vi "Scan Initilize_BU.vi"(4 "Enable DMM Relay":bool=TRUE, 6 "Measure Maximun Voltage":dbl=100.0 format="%#_13g", 7 "Scan Measure\nTime":dbl=17.0, 8 "error in (no error)":errorcluster, 9 "Current Setting":u8[](array[numeric]), 10 "Channel Count":i32, 11 "VISA Refnum in":refnum<visa-resource-name>) -> (0 "error out":errorcluster, 1 "N channel number":i32, 2 "P channel number":i32, 3 "VISA Refnum out":refnum<visa-resource-name>)   [LabVIEW 2023]
uses:
  <instrlib>/Agilent 3446X Series/Agilent 3446X Series.lvlib
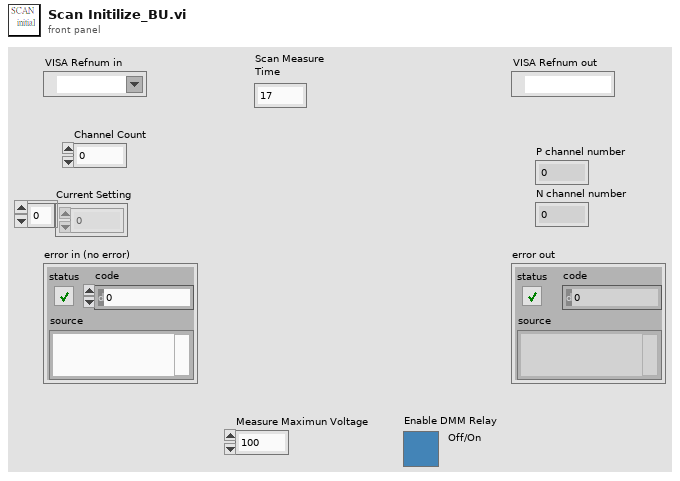
[diagram p1: front panel]
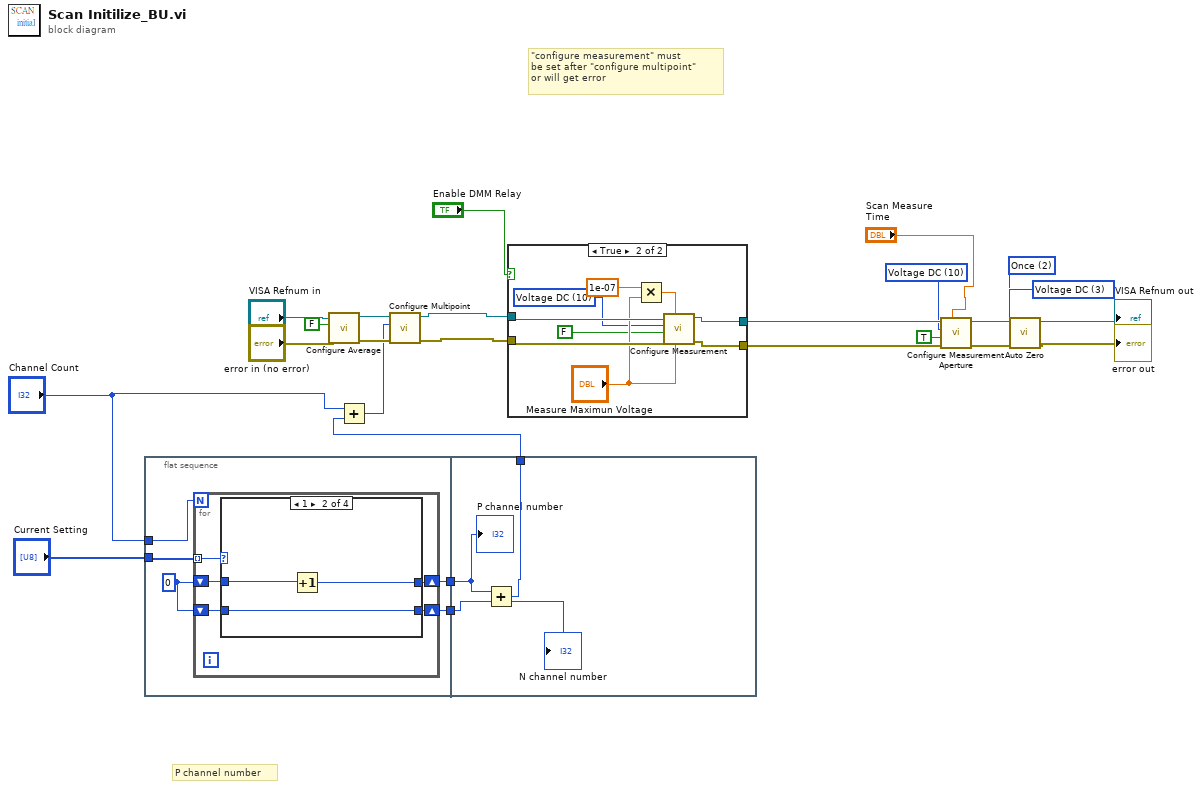
[diagram p0: block diagram]
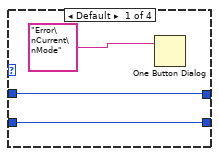
[diagram p3: hidden frame]
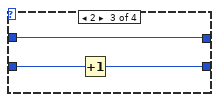
[diagram p4: hidden frame]
diagram:
  w12 = 3 items=["Current DC", "Resistance", "Temperature", "Voltage DC"] ("Zero Type (0: Current DC)")
  w11 = 2 items=["Disable", "Enable", "Once"] ("Auto Zero (1: Enable)")
  w9 = 10 items=["Continuity", "Current AC", "Current DC", "Diode", "Frequency", "Resistance 4-wire", "Period", "Resistance 2-wire", "Temperature", "Voltage AC", "Voltage DC", "Voltage DC Ratio", "Capacitance"] ("Measurement Function (0: Continuity)")
  # "P channel number"
  # "\"configure measurement\" must \nbe set after \"configure multipoint\"\nor will get error"
  n1 = flat-sequence {
    tunnel: "Channel Count" -> [w30]
    tunnel: "Current Setting" -> [w29]
    tunnel: [w27] -> w7
    tunnel: [w26] -> w6
    tunnel: w7 -> [w49]
    tunnel: w6 -> [w48]
    tunnel: [w47] -> w5
    frame #0 {
      w28 = 0 ("P_current_count")
      n2 = for {
        N: w30 -> [_]
        tunnel: w29 -> [w35] mode=indexing
        shift-right: [w33] -> w27
        shift-left: w28 -> [w34]
        shift-right: [w31] -> w26
        shift-left: w28 -> [w32]
        n3 = case shown="1" w35 {
          tunnel: w34 -> [w37 w41 w42 w46]
          tunnel: [w37 w40 w42 w46] -> w33
          tunnel: w32 -> [w36 w39 w44 w45]
          tunnel: [w36 w39 w43 w45] -> w31
          frame Default {
            n4 = One Button Dialog(message="Error\nCurrent\nMode" ("error source (\" \")")) -> ()  [unwired: 1 in, 1 out]
          }
          frame 1 {
            n5 = Increment(x=w41) -> (x+1=w40:i32)
          }
          frame 2 {
            n6 = Increment(x=w44) -> (x+1=w43:i32)
          }
          frame 0 {
          }
        }
      }
    }
    frame #1 {
      n7 = Add(x=w49, y=w48) -> (x+y=w47:i32)
      "P channel number" <- w49
      "N channel number" <- w48
    }
  }
  n8 = call <instrlib>:"Configure Average.vi"("error in (no error)"="error in (no error)", "Enable Statistics (F: Disable)"=FALSE, "VISA resource name"="VISA Refnum in") -> ("error out"=w19:errorcluster, "VISA resource name out"=w18:refnum<visa-resource-name>)  [unwired: 7 in]
  n9 = Add(x="Channel Count", y=w5) -> (x+y=w3:i32)
  n10 = call <instrlib>:"Configure Multipoint.vi"("error in (no error)"=w19, "Trigger Count (1)"=w3, "VISA resource name"=w18) -> ("error out"=w21:errorcluster, "VISA resource name out"=w20:refnum<visa-resource-name>)  [unwired: 4 in, 3 out]
  n11 = case shown="True" "Enable DMM Relay" {
    tunnel: [w50 w60] -> w23
    tunnel: [w51 w59] -> w22
    tunnel: w21 -> [w50 w58]
    tunnel: w20 -> [w51 w57]
    frame False {
    }
    frame True {
      w53 = 10 items=["Continuity", "Current AC", "Current DC", "Diode", "Frequency", "Resistance 4-wire", "Period", "Resistance 2-wire", "Temperature", "Voltage AC", "Voltage DC", "Voltage DC Ratio", "Capacitance"] ("Measurement Function (10: Voltage DC)")
      n12 = Multiply(x=1e-07, y="Measure Maximun Voltage") -> (x*y=w54:dbl)
      n13 = call <instrlib>:"Configure Measurement.vi"("Manual Range (1)"="Measure Maximun Voltage", "Absolute Resolution (1E-6)"=w54, "error in (no error)"=w58, "Auto Range (T: Enable)"=FALSE, "Measurement Function (10: Voltage DC)"=w53, "VISA resource name"=w57) -> ("error out"=w60:errorcluster, "VISA resource name out"=w59:refnum<visa-resource-name>)  [unwired: 4 out]
    }
  }
  n14 = call <instrlib>:"Configure Measurement Aperture.vi"("Aperture Time (0.1s)"="Scan Measure\nTime", "error in (no error)"=w23, "Enable Aperture (F: Disable)"=TRUE, "Measurement Function (0: Continuity)"=w9, "VISA resource name"=w22) -> ("error out"=w13:errorcluster, "VISA resource name out"=w17:refnum<visa-resource-name>)  [unwired: 5 in]
  n15 = call <instrlib>:"Auto Zero.vi"("error in (no error)"=w13, "Auto Zero (1: Enable)"=w11, "Zero Type (0: Current DC)"=w12, "VISA resource name"=w17) -> ("error out"=→"error out":errorcluster, "VISA resource name out"=→"VISA Refnum out":refnum<visa-resource-name>)  [unwired: 6 in]
